vi "Cheesy_Vision.vi"(9 "Smart Dashboard Name":string="CheesyVision", 10 "Settings File":string="CheesyConfig.csv", 11 "Threshold":sgl(knob)=100.0 scale=0.0..200.0) -> ()   [LabVIEW 2015]
uses:
  <vilib>/vision/driver/IMAQdx.llb/IMAQdx Camera Control Mode.ctl
  <vilib>/userdefined/High Color/IMAQdx.ctl
  <vilib>/Utility/file.llb/Read From Spreadsheet File (string).vi
  <vilib>/vision/driver/NI_Vision_Acquisition_Software.lvlib
  <vilib>/vision/NI_Vision_Development_Module.lvlib
panel:
  in  "Save Settings On Exit":bool
  in  "stop":bool
  out "Scores":sgl[](array[numeric])
  out "Different":bool[](array[boolean])
  in  "Region Control":u16(ring) items=["Safe Mode", "Control", "Left", "Right"]
  out "FPS":dbl format="%#_3g"
  out "Image":T1(plugin-control)
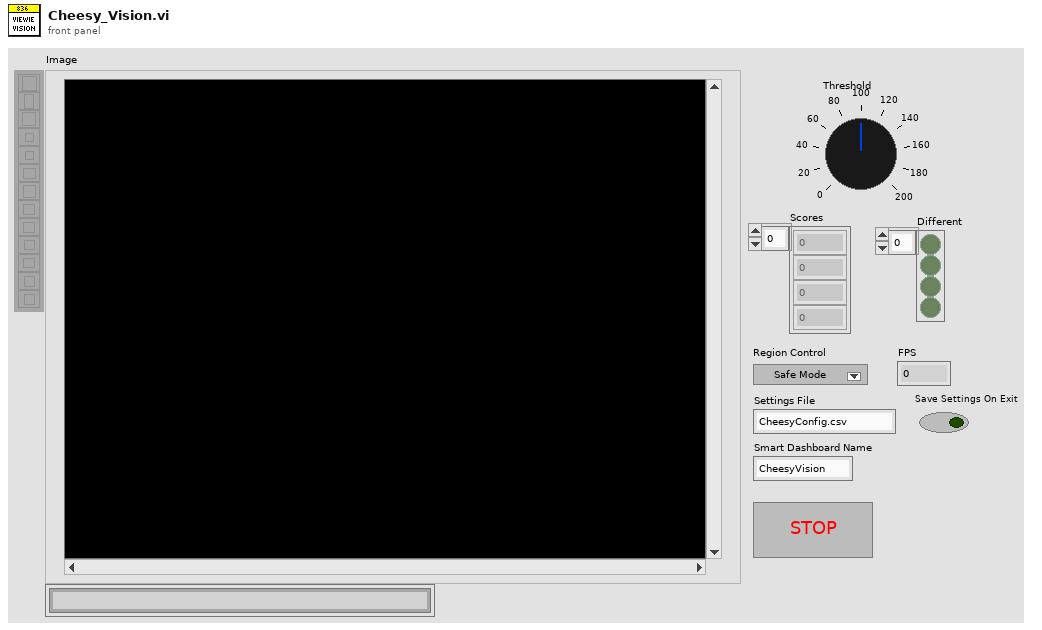
[diagram p1: front panel]
types:
  T1 = typedef "IMAQ Image.ctl" = refnum<image>
  T2 = cluster{"Rectangle Color":u32, "Text Color":u32, "Fill Color":u32}
  T3 = typedef "ROI Descriptor" = cluster{"Global Rectangle":i32[], "Contours":cluster{"ID":enum32{"External", "Internal"}, "Type":u32, "Coordinates":i32[]}[]}
  T4 = typedef "Image Type" = u32
  T5 = typedef "IMAQdx.ctl" = refnum<k21>
  T6 = typedef "NI_Vision_Acquisition_Software.lvlib/IMAQdx Camera Control Mode.ctl" = enum32{"Controller", "Listener"}
  T7 = enum16{"open", "replace", "create", "open or create", "replace or create", "replace or create with confirmation"}
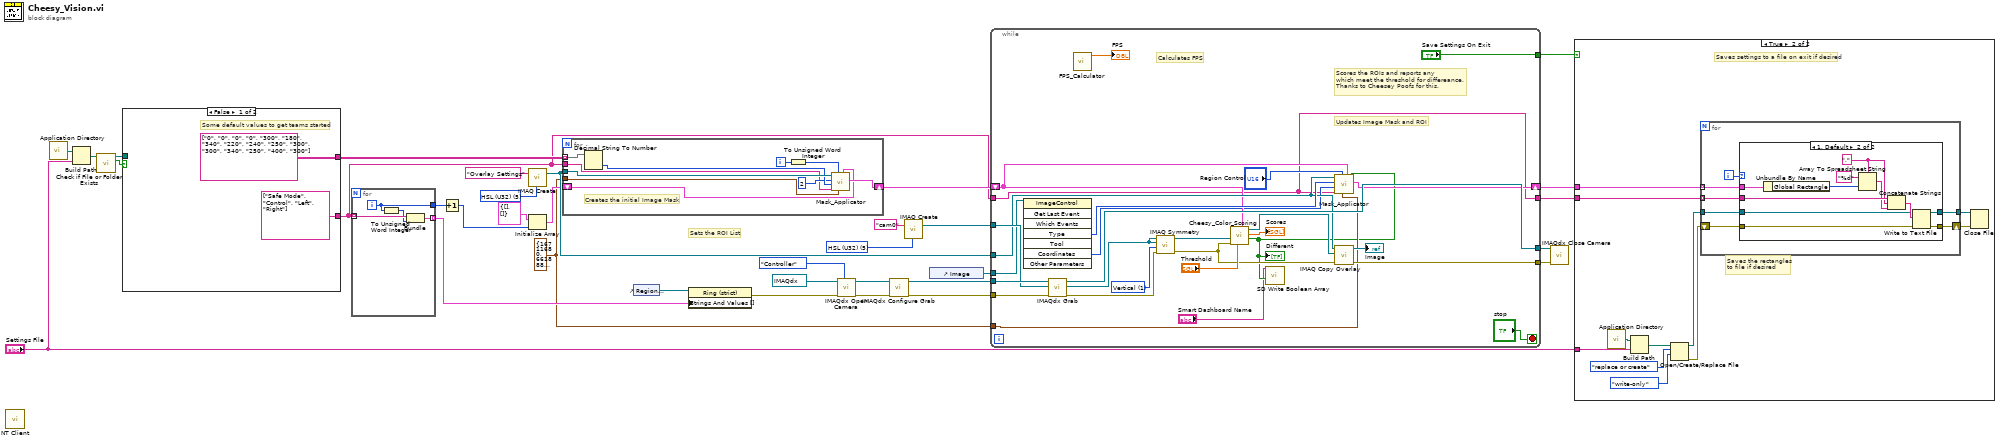
[diagram p0: block diagram]
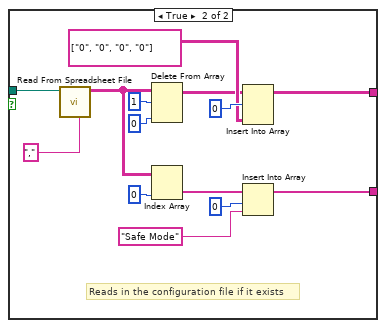
[diagram p2: hidden frame]
diagram:
  w2 = T2 {"Rectangle Color"=16711680, "Text Color"=6618880, "Fill Color"=16776960} ("Cluster")
  w23 = T4 5 items=["Grayscale (U8)", "Grayscale (I16)", "Grayscale (SGL)", "Complex (CSG)", "RGB (U32)", "HSL (U32)", "RGB (U64)", "Grayscale (U16)"] ("Image Type")
  w30 = T4 5 items=["Grayscale (U8)", "Grayscale (I16)", "Grayscale (SGL)", "Complex (CSG)", "RGB (U32)", "HSL (U32)", "RGB (U64)", "Grayscale (U16)"] ("Image Type")
  # "Sets the ROI List"
  n1 = call <vilib>:"NT Client.vi"() -> ()  [unwired: 12 in]
  n2 = call <vilib>:"Application Directory.vi"() -> ("Application Directory"=w14:path)
  n3 = Build Path(base path=w14, name or relative path="Settings File") -> (appended path=w13:path)
  n4 = call <vilib>:"Check if File or Folder Exists.vi"("path"=w13) -> ("file or folder exists?"=w11:bool, "dup path"=w12:path)  [unwired: 8 in, 1 out]
  n5 = case shown="False" w11 {
    tunnel: w12 -> [_ w50]
    tunnel: [string[] ["Safe Mode", "Control", "Left", "Right"] w46] -> w7
    tunnel: [string[][] [["0", "0", "0", "0"], ["300", "180", "340", "220"], ["240", "250", "300", "300"], ["340", "250", "400", "300"]] ("all rows") w41] -> w10
    frame False {
      # "Some default values to get teams started"
    }
    frame True {
      # "Reads in the configuration file if it exists"
      n6 = call-poly <vilib>:"Read From Spreadsheet File.vi"("delimiter (\\t)"="," ("delimiter (\\t)"), "file path (dialog if empty)"=w50) -> ("all rows"=w40:string[][])  [unwired: 5 in, 4 out]
      n7 = Delete From Array(array=w40, length=1, index (col)=0 ("disabled index (col)")) -> (array with subset deleted=w37:string[][])  [unwired: 1 in, 1 out]
      n8 = Index Array(array=w40, index (col)=0 ("disabled index (col)")) -> (element=w47:string[])  [unwired: 1 in]
      n9 = Insert Into Array(array=w37, index (row)=0, new element=string[][] [["0", "0", "0", "0"]] ("all rows")) -> (w41:string[][])  [unwired: 1 in]
      n10 = Insert Into Array(array=w47, index=0, new element="Safe Mode" ("new element/subarray")) -> (w46:string[])
    }
  }
  n11 = for {
    tunnel: w7 -> [w54] mode=indexing
    tunnel: [w53] -> w20 mode=indexing
    tunnel: [w51] -> w3
    i -> [w51]
    n12 = To Unsigned Word Integer(number=w51) -> (unsigned 16bit integer=w52:u16)
    n13 = Bundle("String"=w54, w52) -> (w53:cluster{"String":string, u16})  [unwired: 1 in]
  }
  n14 = Increment(x=w3) -> (x+1=w1:i32)
  n15 = call "IMAQ Create"("Image Name"="Overlay Settings", "Image Type"=w23) -> ("New Image"=w8:T1)  [unwired: 2 in, 2 out]
  n16 = Initialize Array(T3 {"Global Rectangle"=[], "Contours"=[]} ("element"), w1) -> (w4:T3[])
  n17 = for {
    tunnel: w10 -> [w64] mode=indexing
    tunnel: w8 -> [w63]
    shift-right: [w61] -> w9
    shift-left: w4 -> [w60]
    tunnel: w7 -> [w56]
    tunnel: w2 -> [w55]
    i -> [w58]
    # "Creates the initial Image Mask"
    n18 = Decimal String To Number(string=w64) -> (number=w62:i32[])  [unwired: 2 in, 1 out]
    n19 = To Unsigned Word Integer(number=w58) -> (unsigned 16bit integer=w57:u16)
    n20 = call <userlib>:"Mask_Applicator.vi"("ROI In"=w60, "Cluster"=w55, "ROI Number"=w57, "ROI List In"=w56, "Event Coordinates"=w62, "Event Type"=2, "Image Mask"=w63) -> ("ROI Out"=w61:T3[])  [unwired: 3 in, 1 out]
  }
  n21 = control-ref of="Region Control"() -> (w21:refnum<vi>)
  n22 = property on="Property Node" class="Ring (strict)"(reference=w21, "Strings And Values []"=w20) -> (error out=w22:errorcluster)  [unwired: 1 in, 1 out]
  n23 = call <vilib>:"IMAQdx Open Camera.vi"("Camera Control Mode"=IMAQdx_Camera_Control_Mode."Controller", "error in"=w22, "Session In"=T5 "cam0") -> ("error out"=w28:errorcluster, "Session Out"=w18:T5)  [unwired: 7 in]
  n24 = call <vilib>:"IMAQdx Configure Grab.vi"("error in"=w28, "Session In"=w18) -> ("error out"=w26:errorcluster, "Session Out"=w27:T5)  [unwired: 8 in]
  n25 = call "IMAQ Create"("Image Name"="cam0", "Image Type"=w30) -> ("New Image"=w32:T1)  [unwired: 2 in, 2 out]
  n26 = control-ref of="Image"() -> (w25:refnum<vi>)
  n27 = while {
    tunnel: w26 -> [w92]
    tunnel: [w74] -> w34
    tunnel: w27 -> [w90]
    tunnel: [w89] -> w33
    tunnel: w32 -> [w88]
    tunnel: w25 -> [w87]
    tunnel: w8 -> [w84]
    tunnel: w7 -> [w68]
    shift-right: [w83] -> w17
    shift-left: w9 -> [w81]
    tunnel: [w68] -> w16
    tunnel: ["Save Settings On Exit"] -> w15
    tunnel: w2 -> [w67]
    stop <- "stop" stop-if-true
    w79 = u32 1 items=["Horizontal", "Vertical", "Central", "1st Diagonal", "2nd Diagonal"] ("Type of Symmetry")
    # "Calculates FPS"
    # "Scores the ROIs and reports any\nwhich meet the threshold for differeance.\nThanks to Cheesey Poofs for this."
    # "Updates Image Mask and ROI"
    n28 = invoke class="ImageControl" method="Get Last Event"(reference=w87) -> ("Type"=w86:i32, "Coordinates"=w80:i32[])  [unwired: 7 in, 6 out]
    n29 = call <vilib>:"IMAQdx Grab.vi"("error in"=w92, "Image In"=w88, "Session In"=w90) -> ("error out"=w75:errorcluster, "Image Out"=w78:T1, "Session Out"=w89:T5)  [unwired: 5 in, 1 out]
    n30 = call <userlib>:"FPS_Calculator.vi"() -> ("FPS"=→"FPS":dbl)  [unwired: 11 in]
    n31 = call "IMAQ Symmetry"("error in (no error)"=w75, "Type of Symmetry"=w79, "Image Dst"=w78, "Image Src"=w78) -> ("error out"=w69:errorcluster, "Image Dst Out"=w73:T1)  [unwired: 1 in]
    n32 = call <userlib>:"Cheesy_Color_Scoring.vi"("ROI Out"=w81, "Threshold"="Threshold", "error in (no error)"=w69, "Source Image In"=w73) -> ("ROI Different"=w66:bool[], "ROI Scores"=→"Scores":sgl[], "Source Image Out"=w70:T1)  [unwired: 5 in]
    "Different" <- w66
    n33 = call <vilib>:"SD Write Boolean Array.vi"("Boolean Array"=w66, "Name"="Smart Dashboard Name") -> ()  [unwired: 8 in, 2 out]
    n34 = call <userlib>:"Mask_Applicator.vi"("ROI Different"=w66, "ROI In"=w81, "Cluster"=w67, "ROI Number"="Region Control", "ROI List In"=w68, "Event Coordinates"=w80, "Event Type"=w86, "Image Mask"=w84) -> ("ROI Out"=w83:T3[])  [unwired: 2 in, 1 out]
    n35 = call "IMAQ Copy Overlay"("error in (no error)"=w69, "Image Dst"=w70, "Image Src"=w84) -> ("error out"=w74:errorcluster, "Image Dst Out"=→"Image":T1)  [unwired: 7 in]
  }
  n36 = call <vilib>:"IMAQdx Close Camera.vi"("error in"=w34, "Session In"=w33) -> ()  [unwired: 9 in, 1 out]
  n37 = case shown="True" w15 {
    tunnel: w17 -> [_ w103]
    tunnel: w16 -> [_ w102]
    tunnel: "Settings File" -> [_ w93]
    frame False {
    }
    frame True {
      # "Saves settings to a file on exit if desired"
      # "Saves the rectangles\nto file if desired"
      n38 = call <vilib>:"Application Directory.vi"() -> ("Application Directory"=w99:path)
      n39 = Build Path(base path=w99, name or relative path=w93) -> (appended path=w98:path)
      n40 = Open/Create/Replace File(file path (use dialog)=w98, operation (0:open)=T7."replace or create", access (0:read/write)=enum16{"read/write", "read-only", "write-only"}."write-only") -> (refnum out=w97:refnum<file>, error out=w96:errorcluster)  [unwired: 3 in, 1 out]
      n41 = for {
        tunnel: w103 -> [w110] mode=indexing
        tunnel: w102 -> [w109] mode=indexing
        tunnel: w97 -> [w108]
        tunnel: [w106] -> w95
        shift-right: [w105] -> w94
        shift-left: w96 -> [w107]
        i -> [w104]
        n42 = case shown="1, Default" w104 {
          tunnel: w110 -> [_ w123]
          tunnel: w109 -> [_ w120]
          tunnel: w108 -> [w112 w118]
          tunnel: w107 -> [w111 w117]
          tunnel: [w112 w116] -> w106
          tunnel: [w111 w115] -> w105
          frame 0 {
          }
          frame 1, Default {
            w113 = "," ("delimiter (Tab)")
            n43 = Unbundle By Name(w123) -> ("Global Rectangle"=w122:i32[])
            n44 = Array To Spreadsheet String(delimiter (Tab)=w113, array=w122, 3:"%d" ("format string")) -> (spreadsheet string=w114:string)
            n45 = Concatenate Strings(w120, w113, w114) -> (w119:string)
            n46 = Write to Text File(file (use dialog)=w118, text=w119, error in=w117) -> (refnum out=w116:refnum<file>, error out=w115:errorcluster)  [unwired: 1 in, 1 out]
          }
        }
      }
      n47 = Close File(refnum=w95, error in=w94) -> ()  [unwired: 2 out]
    }
  }
